vi "GetOverlay.vi"(8 "error in":errorcluster, 11 "CEF_serializable node in":refnum<class "CEF_serializable node.lvclass">) -> (0 "error out":errorcluster, 2 "overlay":string, 3 "CEF_serializable node out":refnum<class "CEF_serializable node.lvclass">)   [LabVIEW 2023, in "CEF.lvlib" / "CEF_serializable node.lvclass"]
doc: "Copyright 2017 National Instruments Corporation\n\nLicensed under the Apache License, Version 2.0 (the \"License\"); you may not use this file except in compliance with the License. You may obtain a copy of the License at http://www.apache.org/licenses/LICENSE-2.0\nUnless required by applicable law or agreed to in writing, software distributed under the License is distributed on an \"AS IS\" BASIS, WITHOUT WARRANTIES OR CONDITIONS OF ANY KIND, either express or implied. See the License for the specific language governing permissions and limitations under the License."
uses:
  CEF_serializable node.lvclass
  serializable configuration/CEF_serializable configuration.lvclass
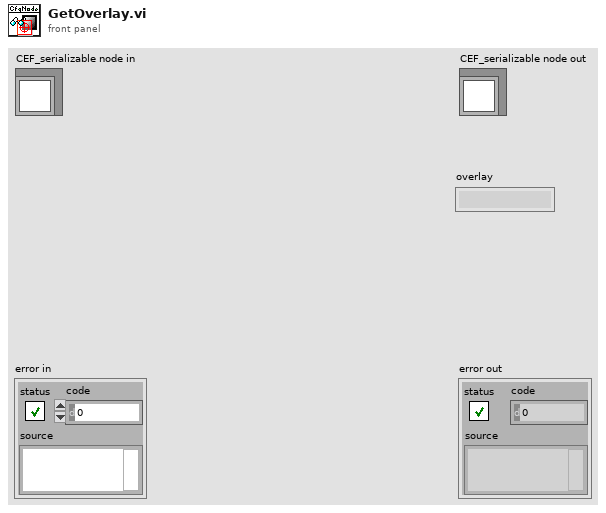
[diagram p1: front panel]
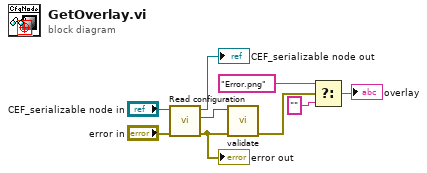
[diagram p0: block diagram]
diagram:
  n1 = call-dynamic "Read configuration.vi"("error in"="error in", "CEF_serializable node in"="CEF_serializable node in") -> ("error out"=w4:errorcluster, "CEF Configuration"=w5:refnum<class "CEF_serializable configuration.lvclass">, "CEF_serializable node out"=→"CEF_serializable node out":refnum<class "CEF_serializable node.lvclass">)  [unwired: 7 in]
  "error out" <- w4
  n2 = call-dynamic "validate.vi"("error in"=w4, "CEF_Configuration in"=w5) -> ("error out"=w3:errorcluster)  [unwired: 8 in, 1 out]
  n3 = Select(t="Error.png", s=w3, f="") -> (s? t:f=→"overlay":string)
